vi "PackedToCart—HexUC,RhomBrav.vi"(1 "Scale mult. ( um )":i32=50, 2 "Packed coordinates ( qword 1D array )":i64[](array[numeric])=[0, 0, 0]) -> (0 "Cartesian coordinates ( double 1D array )":dbl[](array[numeric]))   [LabVIEW 2020]
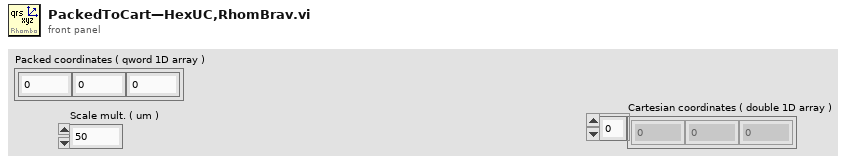
[diagram p1: front panel]
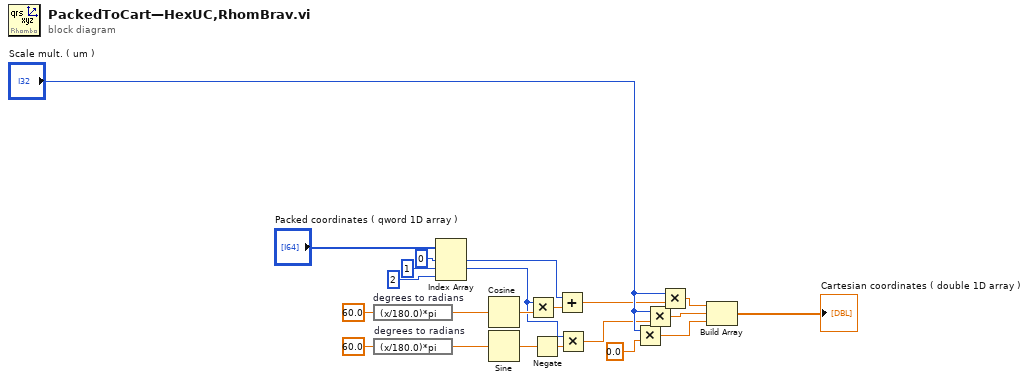
[diagram p0: block diagram]
diagram:
  n1 = expression code="(x/180.0)*pi" "degrees to radians"(60.0) -> (w6:dbl)
  n2 = expression code="(x/180.0)*pi" "degrees to radians"(60.0) -> (w8:dbl)
  n3 = Index Array(array="Packed coordinates ( qword 1D array )", index #1=0 ("index"), index #2=1 ("index"), index #3=2 ("index")) -> (element #1=w22:i64, element #2=w1:i64)  [unwired: 1 out]
  n4 = Cosine(x=w6) -> (cos(x)=w9:dbl)
  n5 = Sine(x=w8) -> (sin(x)=w11:dbl)
  n6 = Multiply(x=w1, y=w9) -> (x*y=w10:dbl)
  n7 = Negate(x=w11) -> (-x=w12:dbl)
  n8 = Add(x=w22, y=w10) -> (x+y=w16:dbl)
  n9 = Multiply(x=w1, y=w12) -> (x*y=w19:dbl)
  n10 = Multiply(x="Scale mult. ( um )", y=0.0 ("element")) -> (x*y=w18:dbl)
  n11 = Multiply(x="Scale mult. ( um )", y=w19) -> (x*y=w17:dbl)
  n12 = Multiply(x="Scale mult. ( um )", y=w16) -> (x*y=w15:dbl)
  n13 = Build Array(w15, w17, w18) -> (→"Cartesian coordinates ( double 1D array )":dbl[])
